vi "Default Entry Value--String.vi"(10 "Theme Control Property":T1, 11 "Window Element":T2) -> (3 "Default Value As String":string)   [LabVIEW 2021, in "Appearance Actor.lvlib" / "Generic Theme.lvclass"]
doc: "For a given <B>Window Element</B> and <B>Theme Control Property</B> pair (Theme Entry), returns the corresponding default value for String entries."
uses:
  Generic Theme.lvclass
  Typedefs/Window Element--enum.ctl
  Typedefs/Theme Control Property--enum.ctl
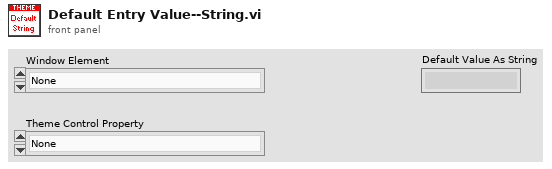
[diagram p1: front panel]
types:
  T1 = typedef "Appearance Actor.lvlib/Generic Theme.lvclass/Theme Control Property--enum.ctl" = enum16{"None", "Button.FalseFillColor", "Button.FalseOutlineColor", "Button.FalseToTrueFillColor", "Button.FalseToTrueOutlineColor", "Button.HoverFalseFillColor", "Button.HoverFalseOutlineColor", "Button.HoverTrueFillColor", "Button.HoverTrueOutlineColor", "Button.TrueFillColor", "Button.TrueOutlineColor", "Button.TrueToFalseFillColor", "Button.TrueToFalseOutlineColor", "CloseButton.FalseFillColor", "CloseButton.FalseOutlineColor", "CloseButton.FalseToTrueFillColor", "CloseButton.FalseToTrueOutlineColor", "CloseButton.HoverFalseFillColor", "CloseButton.HoverFalseOutlineColor", "CloseButton.HoverTrueFillColor", "CloseButton.HoverTrueOutlineColor", "CloseButton.TrueFillColor", "CloseButton.TrueOutlineColor", "CloseButton.TrueToFalseFillColor", "CloseButton.TrueToFalseOutlineColor", "Pane.Color", "Splitter.FillColor", "Splitter.OutlineColor", "Splitter.Size", "Title.Font.Color", "Title.Font.Family", "Title.Font.Size", "Title.Font.Style"}
  T2 = typedef "Appearance Actor.lvlib/Generic Theme.lvclass/Window Element--enum.ctl" = enum16{"None", "TB", "SM", "BP", "SB"}
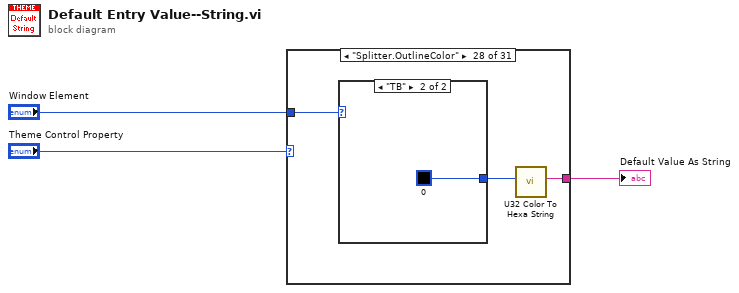
[diagram p0: block diagram]
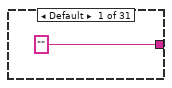
[diagram p2: hidden frame]
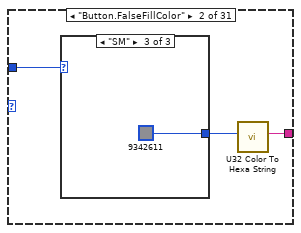
[diagram p3: hidden frame]
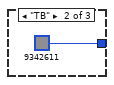
[diagram p5: hidden frame]
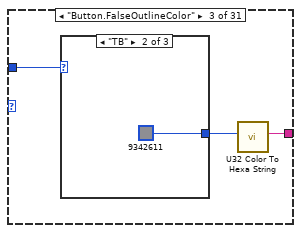
[diagram p6: hidden frame]
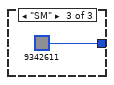
[diagram p8: hidden frame]
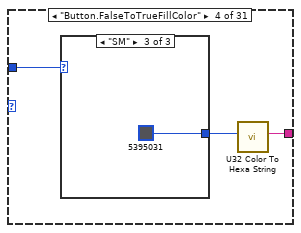
[diagram p9: hidden frame]
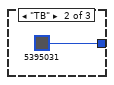
[diagram p11: hidden frame]
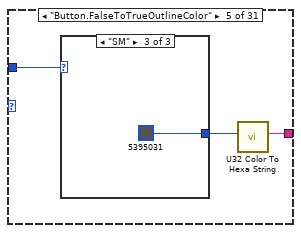
[diagram p12: hidden frame]
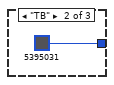
[diagram p14: hidden frame]
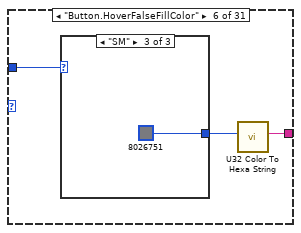
[diagram p15: hidden frame]
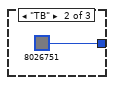
[diagram p17: hidden frame]
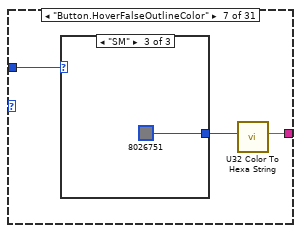
[diagram p18: hidden frame]
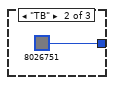
[diagram p20: hidden frame]
diagram:
  n1 = case shown="\"Splitter.OutlineColor\"" "Theme Control Property" {
    tunnel: ["" w7 w12 w17 w22 w27 w32 w37 w42 w47 w52 w57 w62 w67 w71 w75 w79 w83 w87 w91 w95 w99 w103 w107 w111 w115 w122 w126 w130 w133 w136] -> w1
    tunnel: "Window Element" -> [_ w5 w10 w15 w20 w25 w30 w35 w40 w45 w50 w55 w60 w65 w69 w73 w77 w81 w85 w89 w93 w97 w101 w105 w109 w113 w120 w124 w128 w132 w135]
    frame Default {
    }
    frame "Button.FalseFillColor" {
      n2 = case shown="\"SM\"" w5 {
        tunnel: [_ u32 9342611 u32 9342611] -> w6
        frame Default {
        }
        frame "TB" {
        }
        frame "SM" {
        }
      }
      n3 = call "U32 Color To Hexa String.vi"("U32 Color"=w6) -> ("8 Char Hexa String"=w7:string)  [unwired: 10 in]
    }
    frame "Button.FalseOutlineColor" {
      n4 = case shown="\"TB\"" w10 {
        tunnel: [_ u32 9342611 u32 9342611] -> w11
        frame Default {
        }
        frame "TB" {
        }
        frame "SM" {
        }
      }
      n5 = call "U32 Color To Hexa String.vi"("U32 Color"=w11) -> ("8 Char Hexa String"=w12:string)  [unwired: 10 in]
    }
    frame "Button.FalseToTrueFillColor" {
      n6 = case shown="\"SM\"" w15 {
        tunnel: [_ u32 5395031 u32 5395031] -> w16
        frame Default {
        }
        frame "TB" {
        }
        frame "SM" {
        }
      }
      n7 = call "U32 Color To Hexa String.vi"("U32 Color"=w16) -> ("8 Char Hexa String"=w17:string)  [unwired: 10 in]
    }
    frame "Button.FalseToTrueOutlineColor" {
      n8 = case shown="\"SM\"" w20 {
        tunnel: [_ u32 5395031 u32 5395031] -> w21
        frame Default {
        }
        frame "TB" {
        }
        frame "SM" {
        }
      }
      n9 = call "U32 Color To Hexa String.vi"("U32 Color"=w21) -> ("8 Char Hexa String"=w22:string)  [unwired: 10 in]
    }
    frame "Button.HoverFalseFillColor" {
      n10 = case shown="\"SM\"" w25 {
        tunnel: [_ u32 8026751 u32 8026751] -> w26
        frame Default {
        }
        frame "TB" {
        }
        frame "SM" {
        }
      }
      n11 = call "U32 Color To Hexa String.vi"("U32 Color"=w26) -> ("8 Char Hexa String"=w27:string)  [unwired: 10 in]
    }
    frame "Button.HoverFalseOutlineColor" {
      n12 = case shown="\"SM\"" w30 {
        tunnel: [_ u32 8026751 u32 8026751] -> w31
        frame Default {
        }
        frame "TB" {
        }
        frame "SM" {
        }
      }
      n13 = call "U32 Color To Hexa String.vi"("U32 Color"=w31) -> ("8 Char Hexa String"=w32:string)  [unwired: 10 in]
    }
    frame "Button.HoverTrueFillColor" {
      n14 = case shown="\"SM\"" w35 {
        tunnel: [_ u32 5395031 u32 5395031] -> w36
        frame Default {
        }
        frame "TB" {
        }
        frame "SM" {
        }
      }
      n15 = call "U32 Color To Hexa String.vi"("U32 Color"=w36) -> ("8 Char Hexa String"=w37:string)  [unwired: 10 in]
    }
    frame "Button.HoverTrueOutlineColor" {
      n16 = case shown="\"SM\"" w40 {
        tunnel: [_ u32 5395031 u32 5395031] -> w41
        frame Default {
        }
        frame "TB" {
        }
        frame "SM" {
        }
      }
      n17 = call "U32 Color To Hexa String.vi"("U32 Color"=w41) -> ("8 Char Hexa String"=w42:string)  [unwired: 10 in]
    }
    frame "Button.TrueFillColor" {
      n18 = case shown="\"SM\"" w45 {
        tunnel: [_ u32 6710891 u32 6710891] -> w46
        frame Default {
        }
        frame "TB" {
        }
        frame "SM" {
        }
      }
      n19 = call "U32 Color To Hexa String.vi"("U32 Color"=w46) -> ("8 Char Hexa String"=w47:string)  [unwired: 10 in]
    }
    frame "Button.TrueOutlineColor" {
      n20 = case shown="\"SM\"" w50 {
        tunnel: [_ u32 6710891 u32 6710891] -> w51
        frame Default {
        }
        frame "TB" {
        }
        frame "SM" {
        }
      }
      n21 = call "U32 Color To Hexa String.vi"("U32 Color"=w51) -> ("8 Char Hexa String"=w52:string)  [unwired: 10 in]
    }
    frame "Button.TrueToFalseFillColor" {
      n22 = case shown="\"SM\"" w55 {
        tunnel: [_ u32 8026751 u32 8026751] -> w56
        frame Default {
        }
        frame "TB" {
        }
        frame "SM" {
        }
      }
      n23 = call "U32 Color To Hexa String.vi"("U32 Color"=w56) -> ("8 Char Hexa String"=w57:string)  [unwired: 10 in]
    }
    frame "Button.TrueToFalseOutlineColor" {
      n24 = case shown="\"SM\"" w60 {
        tunnel: [_ u32 8026751 u32 8026751] -> w61
        frame Default {
        }
        frame "TB" {
        }
        frame "SM" {
        }
      }
      n25 = call "U32 Color To Hexa String.vi"("U32 Color"=w61) -> ("8 Char Hexa String"=w62:string)  [unwired: 10 in]
    }
    frame "CloseButton.FalseFillColor" {
      n26 = case shown="\"TB\"" w65 {
        tunnel: [_ u32 9342611] -> w66
        frame Default {
        }
        frame "TB" {
        }
      }
      n27 = call "U32 Color To Hexa String.vi"("U32 Color"=w66) -> ("8 Char Hexa String"=w67:string)  [unwired: 10 in]
    }
    frame "CloseButton.FalseOutlineColor" {
      n28 = case shown="\"TB\"" w69 {
        tunnel: [_ u32 9342611] -> w70
        frame Default {
        }
        frame "TB" {
        }
      }
      n29 = call "U32 Color To Hexa String.vi"("U32 Color"=w70) -> ("8 Char Hexa String"=w71:string)  [unwired: 10 in]
    }
    frame "CloseButton.FalseToTrueFillColor" {
      n30 = case shown="\"TB\"" w73 {
        tunnel: [_ u32 12011595] -> w74
        frame Default {
        }
        frame "TB" {
        }
      }
      n31 = call "U32 Color To Hexa String.vi"("U32 Color"=w74) -> ("8 Char Hexa String"=w75:string)  [unwired: 10 in]
    }
    frame "CloseButton.FalseToTrueOutlineColor" {
      n32 = case shown="\"TB\"" w77 {
        tunnel: [_ u32 12011595] -> w78
        frame Default {
        }
        frame "TB" {
        }
      }
      n33 = call "U32 Color To Hexa String.vi"("U32 Color"=w78) -> ("8 Char Hexa String"=w79:string)  [unwired: 10 in]
    }
    frame "CloseButton.HoverFalseFillColor" {
      n34 = case shown="\"TB\"" w81 {
        tunnel: [_ u32 12856092] -> w82
        frame Default {
        }
        frame "TB" {
        }
      }
      n35 = call "U32 Color To Hexa String.vi"("U32 Color"=w82) -> ("8 Char Hexa String"=w83:string)  [unwired: 10 in]
    }
    frame "CloseButton.HoverFalseOutlineColor" {
      n36 = case shown="\"TB\"" w85 {
        tunnel: [_ u32 12856092] -> w86
        frame Default {
        }
        frame "TB" {
        }
      }
      n37 = call "U32 Color To Hexa String.vi"("U32 Color"=w86) -> ("8 Char Hexa String"=w87:string)  [unwired: 10 in]
    }
    frame "CloseButton.HoverTrueFillColor" {
      n38 = case shown="\"TB\"" w89 {
        tunnel: [_ u32 14221312] -> w90
        frame Default {
        }
        frame "TB" {
        }
      }
      n39 = call "U32 Color To Hexa String.vi"("U32 Color"=w90) -> ("8 Char Hexa String"=w91:string)  [unwired: 10 in]
    }
    frame "CloseButton.HoverTrueOutlineColor" {
      n40 = case shown="\"TB\"" w93 {
        tunnel: [_ u32 14221312] -> w94
        frame Default {
        }
        frame "TB" {
        }
      }
      n41 = call "U32 Color To Hexa String.vi"("U32 Color"=w94) -> ("8 Char Hexa String"=w95:string)  [unwired: 10 in]
    }
    frame "CloseButton.TrueFillColor" {
      n42 = case shown="\"TB\"" w97 {
        tunnel: [_ u32 16711680] -> w98
        frame Default {
        }
        frame "TB" {
        }
      }
      n43 = call "U32 Color To Hexa String.vi"("U32 Color"=w98) -> ("8 Char Hexa String"=w99:string)  [unwired: 10 in]
    }
    frame "CloseButton.TrueOutlineColor" {
      n44 = case shown="\"TB\"" w101 {
        tunnel: [_ u32 16711680] -> w102
        frame Default {
        }
        frame "TB" {
        }
      }
      n45 = call "U32 Color To Hexa String.vi"("U32 Color"=w102) -> ("8 Char Hexa String"=w103:string)  [unwired: 10 in]
    }
    frame "CloseButton.TrueToFalseFillColor" {
      n46 = case shown="\"TB\"" w105 {
        tunnel: [_ u32 12011595] -> w106
        frame Default {
        }
        frame "TB" {
        }
      }
      n47 = call "U32 Color To Hexa String.vi"("U32 Color"=w106) -> ("8 Char Hexa String"=w107:string)  [unwired: 10 in]
    }
    frame "CloseButton.TrueToFalseOutlineColor" {
      n48 = case shown="\"TB\"" w109 {
        tunnel: [_ u32 12011595] -> w110
        frame Default {
        }
        frame "TB" {
        }
      }
      n49 = call "U32 Color To Hexa String.vi"("U32 Color"=w110) -> ("8 Char Hexa String"=w111:string)  [unwired: 10 in]
    }
    frame "Pane.Color" {
      n50 = case shown="\"BP\"" w113 {
        tunnel: [_ u32 9342611 u32 9342611 u32 16448250 u32 9342611] -> w114
        frame Default {
        }
        frame "TB" {
        }
        frame "SM" {
        }
        frame "BP" {
        }
        frame "SB" {
        }
      }
      n51 = call "U32 Color To Hexa String.vi"("U32 Color"=w114) -> ("8 Char Hexa String"=w115:string)  [unwired: 10 in]
    }
    frame "Splitter.FillColor" {
      n52 = case shown="\"TB\"" w120 {
        tunnel: [_ u32 0] -> w121
        frame Default {
        }
        frame "TB" {
        }
      }
      n53 = call "U32 Color To Hexa String.vi"("U32 Color"=w121) -> ("8 Char Hexa String"=w122:string)  [unwired: 10 in]
    }
    frame "Splitter.OutlineColor" {
      n54 = case shown="\"TB\"" w124 {
        tunnel: [_ u32 0] -> w125
        frame Default {
        }
        frame "TB" {
        }
      }
      n55 = call "U32 Color To Hexa String.vi"("U32 Color"=w125) -> ("8 Char Hexa String"=w126:string)  [unwired: 10 in]
    }
    frame "Title.Font.Color" {
      n56 = case shown="\"TB\"" w128 {
        tunnel: [_ u32 16448250] -> w129
        frame Default {
        }
        frame "TB" {
        }
      }
      n57 = call "U32 Color To Hexa String.vi"("U32 Color"=w129) -> ("8 Char Hexa String"=w130:string)  [unwired: 10 in]
    }
    frame "Title.Font.Family" {
      n58 = case shown="\"TB\"" w132 {
        tunnel: [_ "Arial"] -> w133
        frame Default {
        }
        frame "TB" {
        }
      }
    }
    frame "Title.Font.Style" {
      n59 = case shown="\"TB\"" w135 {
        tunnel: [_ "bi"] -> w136
        frame Default {
        }
        frame "TB" {
        }
      }
    }
  }
  "Default Value As String" <- w1
